vi "TIO Device Tick.vi"(8 "Error in":errorcluster, 10 "TIO State":T2={"Awaiting REP"=FALSE, "REQ ID"=500, "dstreams in"=[], "pstreams"=[], "timebases"=[]}, 11 "TIO":T3={"TC Connection"={"Type"=enum."Serial", "URL"="serial:///dev/cu.usbserial-00000", "TO"=500, "Addr"=0, "Port"=0, "TCP"=refnum, "UDP"=refnum, "Route"=""}, "REQ"=refnum, "REP"=refnum}) -> (0 "Error out":errorcluster={"status"=TRUE, "code"=-1073807252, "source"="VISA Read in SLIP Decode Serial Read.vi->NN VISA Read.vi->NN RPC.vi"}, 1 "Data Out":T1, 2 "TIO State":T2={"Awaiting REP"=FALSE, "REQ ID"=500, "dstreams in"=[], "pstreams"=[], "timebases"=[]}, 3 "TIO":T3={"TC Connection"={"Type"=enum."Serial", "URL"="serial:///dev/cu.usbserial-00000", "TO"=500, "Addr"=0, "Port"=0, "TCP"=refnum, "UDP"=refnum, "Route"=""}, "REQ"=refnum, "REP"=refnum})   [LabVIEW 2010]
panel:
  out "Last Log":string
  # "TIO Tick"
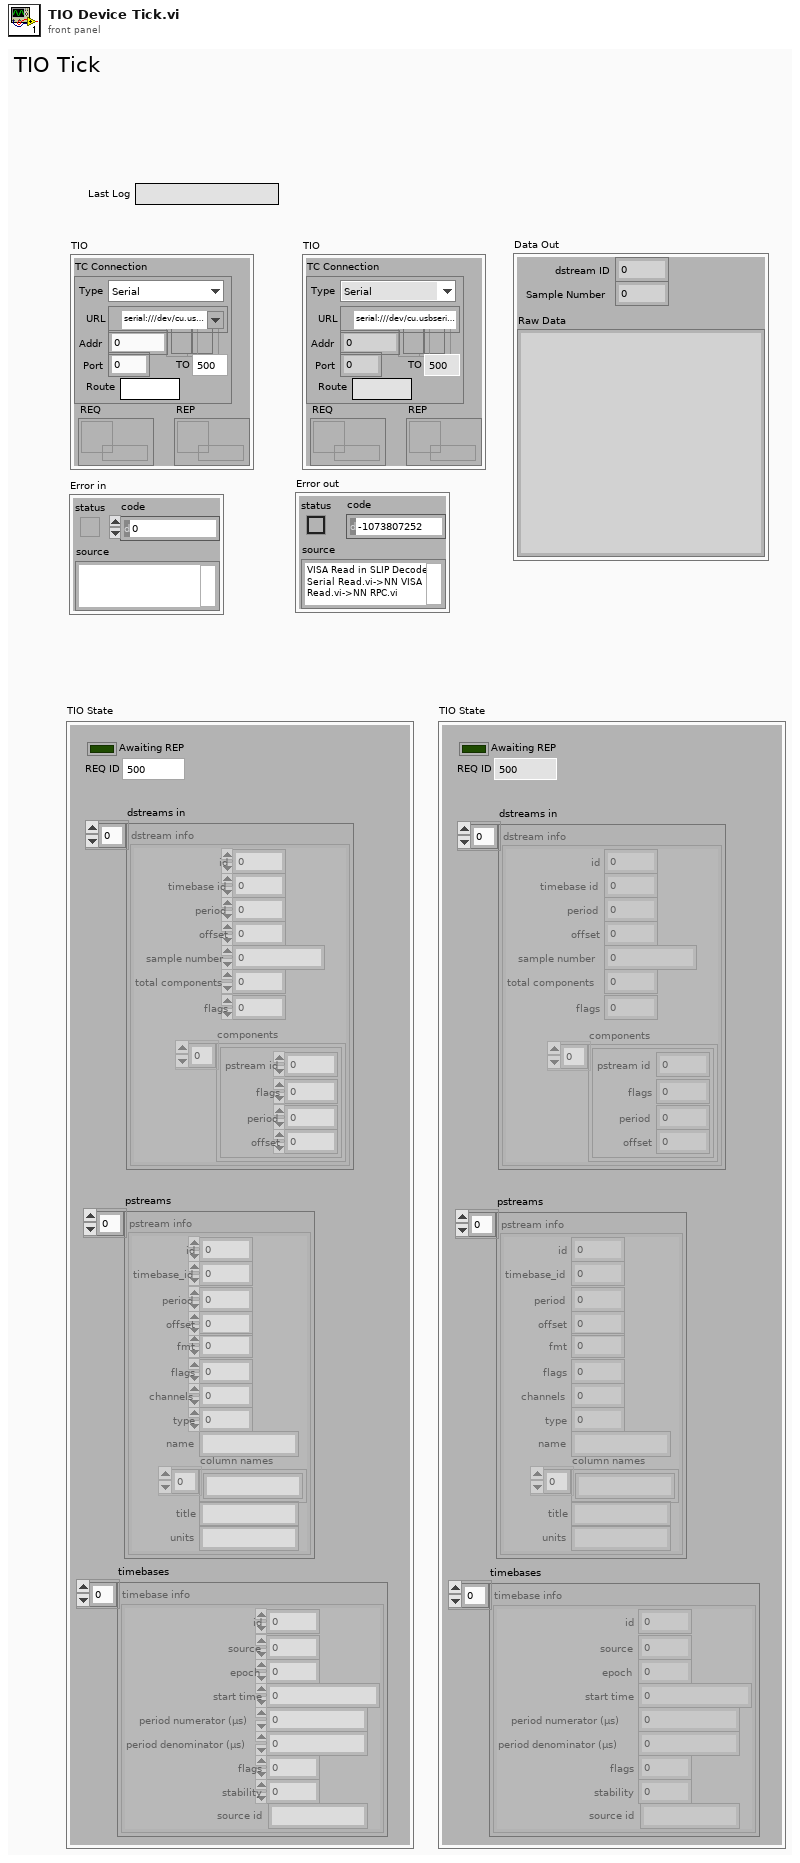
[diagram p1: front panel]
types:
  T1 = cluster{"dstream ID":u16, "Sample Number":u32, "Raw Data":string}
  T2 = cluster{"Awaiting REP":bool, "REQ ID":u32, "dstreams in":cluster{"id":u16, "timebase id":u16, "period":u32, "offset":u32, "sample number":u64, "total components":u16, "flags":u16, "components":cluster{"pstream id":u16, "flags":u16, "period":u32, "offset":u32}[]}[], "pstreams":cluster{"id":u16, "timebase_id":u16, "period":u32, "offset":u32, "fmt":i32, "flags":u16, "channels":u16, "type":u8, "name":string, "column names":string[], "title":string, "units":string}[], "timebases":cluster{"id":u16, "source":u8, "epoch":u8, "start time":u64, "period numerator (µs)":u32, "period denominator (µs)":u32, "flags":u32, "stability":sgl, "source id":string}[]}
  T3 = cluster{"TC Connection":cluster{"Type":enum16{"Serial", "TCP", "UDP", "mUDP"}, "URL":refnum<visa-resource-name>, "TO":u32, "Addr":u32, "Port":i32, "TCP":refnum<k5>, "UDP":refnum<k16>, "Route":string}, "REQ":refnum<queue>, "REP":refnum<queue>}
  T4 = cluster{"Type":enum16{"Serial", "TCP", "UDP", "mUDP"}, "URL":refnum<visa-resource-name>, "TO":u32, "Addr":u32, "Port":i32, "TCP":refnum<k5>, "UDP":refnum<k16>, "Route":string}
  T5 = enum16{"big-endian, network order", "native, host order", "little-endian"}
  T6 = cluster{"id":u16, "source":u8, "epoch":u8, "start time":u64, "period numerator (µs)":u32, "period denominator (µs)":u32, "flags":u32, "stability":sgl, "source id":string}[]
  T7 = cluster{"id":u16, "timebase_id":u16, "period":u32, "offset":u32, "fmt":i32, "flags":u16, "channels":u16, "type":u8, "name":string, "column names":string[], "title":string, "units":string}[]
  T8 = cluster{"id":u16, "timebase_id":u16, "period":u32, "offset":u32, "fmt":i32, "flags":u16, "channels":u16, "type":u8, "name":string, string[], "title":string, "units":string}[]
  T9 = cluster{"id":u16, "timebase id":u16, "period":u32, "offset":u32, "sample number":u64, "total components":u16, "flags":u16, "components":cluster{"pstream id":u16, "flags":u16, "period":u32, "offset":u32}[]}[]
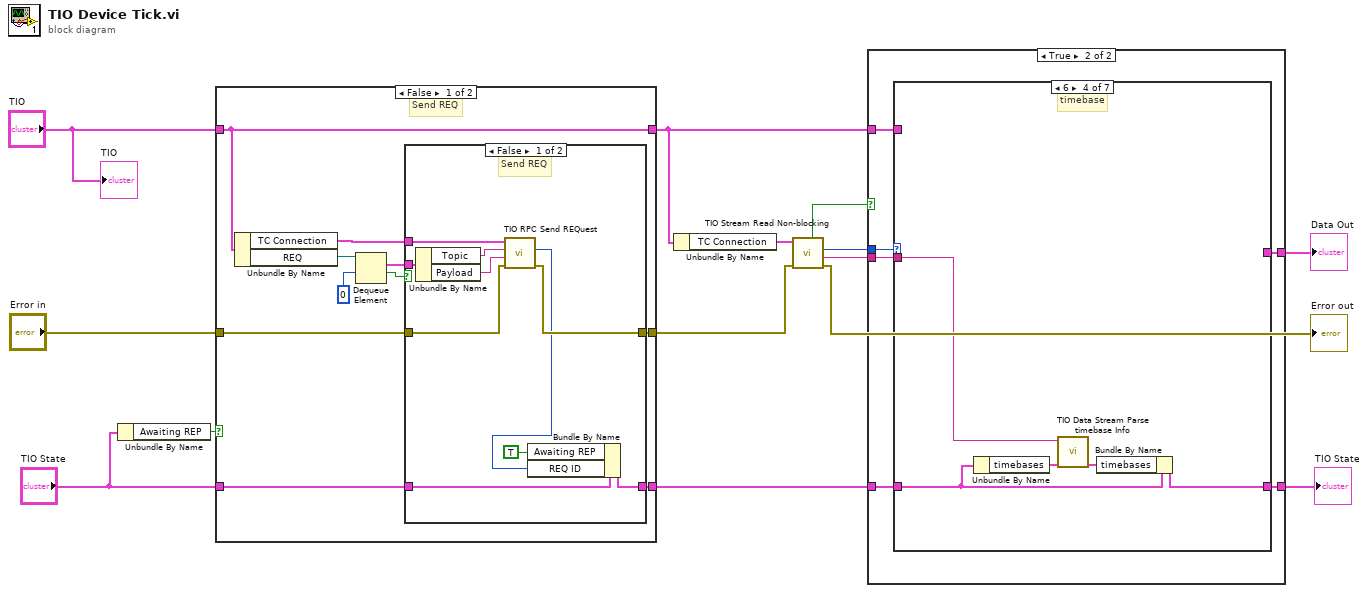
[diagram p0: block diagram]
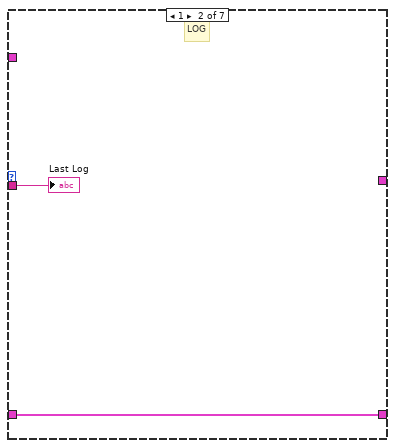
[diagram p4: hidden frame]
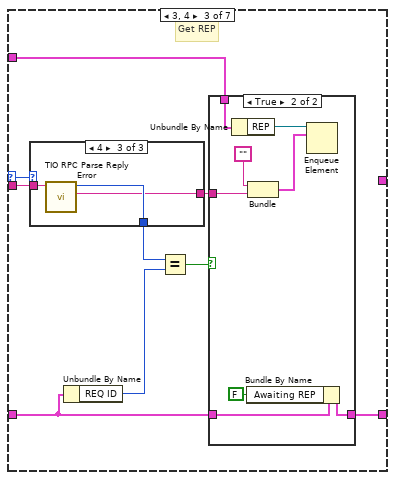
[diagram p5: hidden frame]
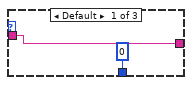
[diagram p6: hidden frame]
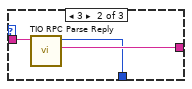
[diagram p7: hidden frame]
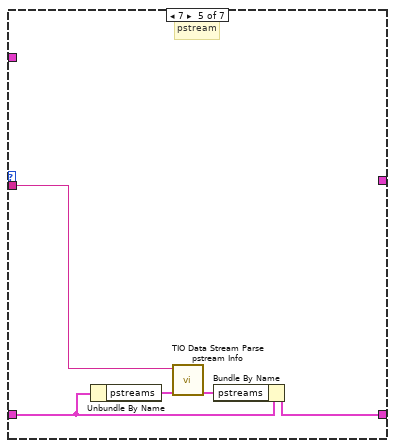
[diagram p9: hidden frame]
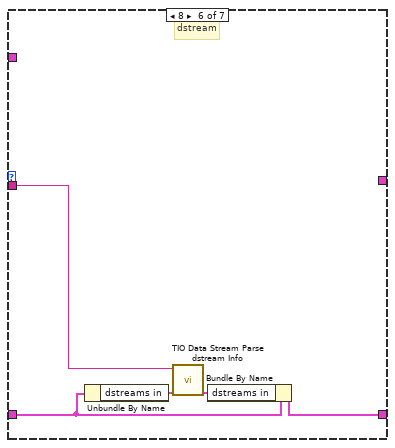
[diagram p10: hidden frame]
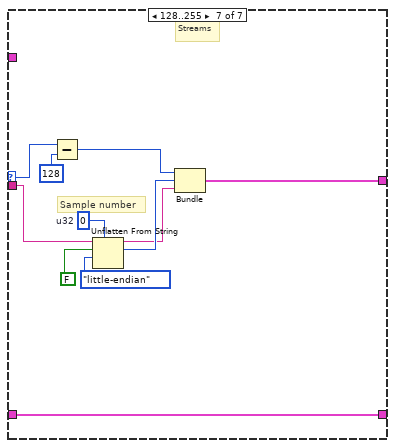
[diagram p11: hidden frame]
diagram:
  n1 = Unbundle By Name("TIO State") -> ("Awaiting REP"=w8:bool)
  n2 = case shown="False" w8 {
    tunnel: [w24 w37] -> w11
    tunnel: [w20 w39] -> w6
    tunnel: "TIO" -> [w20 w39]
    tunnel: "TIO State" -> [w16 w38]
    tunnel: [w17 w38] -> w7
    tunnel: "Error in" -> [w15 w37]
    frame False {
      # "Send REQ"
      n3 = Unbundle By Name(w20) -> ("TC Connection"=w19:T4, "REQ"=w18:refnum<queue>)
      n4 = Dequeue Element(queue=w18, timeout in ms (-1)=0) -> (element=w22:cluster{"Topic":string, "Payload":string}, timed out?=w21:bool)  [unwired: 1 in, 2 out]
      n5 = case shown="False" w21 {
        tunnel: [w34 w35] -> w24
        tunnel: w19 -> [w33 _]
        tunnel: w22 -> [w31 _]
        tunnel: [w28 w36] -> w17
        tunnel: w16 -> [w29 w36]
        tunnel: w15 -> [w26 w35]
        frame False {
          # "Send REQ"
          n6 = Unbundle By Name(w31) -> ("Topic"=w30:string, "Payload"=w32:string)
          n7 = call "TIO RPC Send REQuest.vi"("error in (no error)"=w26, "Payload"=w32, "Topic"=w30, "TC Connection"=w33) -> ("error out"=w34:errorcluster, "Request ID"=w25:u16)  [unwired: 5 in, 1 out]
          n8 = Bundle By Name(cluster=w29, "Awaiting REP"=TRUE, "REQ ID"=w25) -> (w28:T2)
        }
        frame True {
          # "REQ Notification timeout"
        }
      }
    }
    frame True {
      # "Awaiting REP"
    }
  }
  n9 = Unbundle By Name(w6) -> ("TC Connection"=w5:T4)
  n10 = call "TIO Stream Read Non-blocking.vi"("error in (no error)"=w11, "TC Connection"=w5) -> ("error out"=→"Error out":errorcluster, "Payload"=w9:string, "Type"=w10:u16, "Routing Matches"=w1:bool)  [unwired: 4 in, 2 out]
  n11 = case shown="True" w1 {
    tunnel: w10 -> [_ w46]
    tunnel: w9 -> [_ w45]
    tunnel: w7 -> [w40 w44]
    tunnel: w6 -> [_ w43]
    tunnel: [w40 w42] -> w3
    tunnel: [_ w41] -> w2
    frame False {
    }
    frame True {
      n12 = case shown="6" w46 {
        selector: w46 -> [_ _ w50 _ _ _ w101]
        tunnel: w45 -> [_ w49 w58 w78 w83 w90 w93]
        tunnel: w43 -> [_ _ w51 _ _ _ _]
        tunnel: [w47 w48 w52 w79 w84 w88 w99] -> w42
        tunnel: w44 -> [w47 w48 w53 w80 w85 w89 w99]
        tunnel: [_ _ _ _ _ _ w97] -> w41
        frame 0, Default {
        }
        frame 1 {
          # "LOG"
          "Last Log" <- w49
        }
        frame 3, 4 {
          # "Get REP"
          n13 = case shown="4" w50 {
            tunnel: w58 -> [w60 w63 w66]
            tunnel: [w60 w62 w64] -> w57
            tunnel: [u16 0 ("Request ID") w61 w65] -> w55
            frame Default {
            }
            frame 3 {
              n14 = call "TIO RPC Parse Reply.vi"("Payload"=w63) -> ("Payload"=w62:string, "Request ID"=w61:u16)  [unwired: 9 in]
            }
            frame 4 {
              n15 = call "TIO RPC Parse Reply Error.vi"("Payload"=w66) -> ("Payload"=w64:string, "Request ID"=w65:u16)  [unwired: 8 in, 1 out]
            }
          }
          n16 = Unbundle By Name(w53) -> ("REQ ID"=w54:u32)
          n17 = Equal?(x=w55, y=w54) -> (x = y?=w56:bool)
          n18 = case shown="True" w56 {
            tunnel: w57 -> [_ w70]
            tunnel: w53 -> [w67 w75]
            tunnel: [w67 w74] -> w52
            tunnel: w51 -> [_ w73]
            frame False {
            }
            frame True {
              n19 = Unbundle By Name(w73) -> ("REP"=w72:refnum<queue>)
              n20 = Bundle By Name(cluster=w75, "Awaiting REP"=FALSE) -> (w74:T2)
              n21 = Bundle("", "Payload"=w70) -> (w71:cluster{string, "Payload":string})  [unwired: 1 in]
              n22 = Enqueue Element(queue=w72, element=w71) -> ()  [unwired: 2 in, 3 out]
            }
          }
        }
        frame 6 {
          # "timebase"
          n23 = Unbundle By Name(w80) -> ("timebases"=w77:T6)
          n24 = call "TIO Data Stream Parse timebase Info.vi"("timebases in"=w77, "timebase info raw"=w78) -> ("timebases out"=w76:T6)  [unwired: 9 in]
          n25 = Bundle By Name(cluster=w80, "timebases"=w76) -> (w79:T2)
        }
        frame 7 {
          # "pstream"
          n26 = Unbundle By Name(w85) -> ("pstreams"=w82:T7)
          n27 = call "TIO Data Stream Parse pstream Info.vi"("pstreams in"=w82, "pstream info raw"=w83) -> ("pstreams out"=w81:T8)  [unwired: 9 in]
          n28 = Bundle By Name(cluster=w85, "pstreams"=w81) -> (w84:T2)
        }
        frame 8 {
          # "dstream"
          n29 = Unbundle By Name(w89) -> ("dstreams in"=w87:T9)
          n30 = call "TIO Data Stream Parse dstream Info.vi"("dstreams in"=w87, "dstream info raw"=w90) -> ("dstreams in"=w86:T9)  [unwired: 8 in, 1 out]
          n31 = Bundle By Name(cluster=w89, "dstreams in"=w86) -> (w88:T2)
        }
        frame 128..255 {
          w94 = u32 0  # u32
          # "Sample number"
          # "Streams"
          n32 = Subtract(x=w101, y=u16 128) -> (x-y=w98:u16)
          n33 = Unflatten From String(type=w94, binary string=w93, data includes array or string size? (T)=FALSE, byte order (0:big-endian, network order)=T5."little-endian") -> (rest of the binary string=w91:string, value=w92:u32)  [unwired: 1 in, 1 out]
          n34 = Bundle(w98, "u32"=w92, w91) -> (w97:cluster{u16, "u32":u32, string})  [unwired: 1 in]
        }
      }
    }
  }
  "TIO State" <- w3
  "Data Out" <- w2
  "TIO" <- "TIO"
